vi "Arrange.vi"(6 "Variant in":variant, 7 "Shift Pressed?":bool, 8 "error in (no error)":errorcluster, 10 "QD Combo Box Ref":refnum<vi>, 11 "QD Launch VI Ref":refnum<vi>) -> (0 "error out":errorcluster, 4 "Variant out":variant)   [LabVIEW 2019]
doc: "Arranges the block diagram or front panel objects depending on the selection:\n\nFP + No Selection:\n Arranges all controls and indicators by relative position, snaps to grid and resets the panel origins.\n\nFP + Selection:\n Arranges the selected controls by the left edge and snaps to grid. \n Hold Shift to arrange the selected controls by the top edge.\n\nBD + No Selection:\n Arranges all terminals to the adjacent terminal and align controls/indicators left/right respectively.\n\nBD + Selection:\n Arranges the selected objects to adjacent terminal (left-to-right). \n Hold Shift to arrange the selection in reverse order (right-to-left).\n Note: Constants are arranged relative to the adjacent terminal position.\n\nCreated by: Ryan Pacini\n\nDefault Shortcut - [A]"
uses:
  _Script/support/_builtins_arrange.ctl
  _Script/support/Script.lvlib
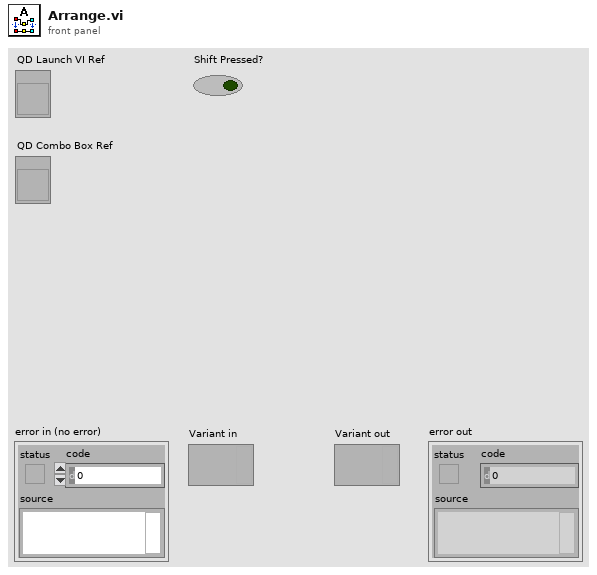
[diagram p1: front panel]
types:
  T1 = typedef "Script.lvlib/_builtins_arrange.ctl" = enum8{"left_to_right", "right_to_left"}
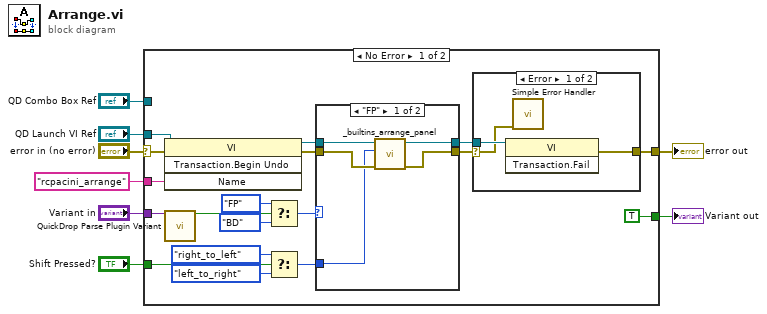
[diagram p0: block diagram]
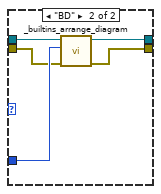
[diagram p2: hidden frame]
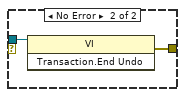
[diagram p3: hidden frame]
diagram:
  n1 = case shown="No Error" "error in (no error)" {
    selector: "error in (no error)" -> [w26 w42]
    tunnel: [w25 w42] -> w3
    tunnel: "QD Launch VI Ref" -> [w21 _]
    tunnel: "rcpacini_arrange" ("Undo Name") -> [w24 _]
    tunnel: "Variant in" -> [w22 _]
    tunnel: [TRUE _] -> w4
    tunnel: "QD Combo Box Ref" -> [_ _]
    tunnel: "Shift Pressed?" -> [w16 _]
    frame No Error {
      n2 = invoke class="VI" method="Transaction.Begin Undo"(reference=w21, error in=w26, "Name"=w24) -> (reference out=w20:refnum<vi>, error out=w19:errorcluster)  [unwired: 1 in, 2 out]
      n3 = call <vilib>:"QuickDrop Parse Plugin Variant.vi"("QDKS Variant in"=w22) -> ("QD Launch VI Panel?"=w12:bool)  [unwired: 12 in, 2 out]
      n4 = Select(t=enum8{"FP", "BD"}."FP" ("Panel"), s=w12, f=enum8{"FP", "BD"}."BD" ("Panel")) -> (s? t:f=w11:enum8{"FP", "BD"})
      n5 = Select(t=_builtins_arrange."right_to_left" ("Arrange"), s=w16, f=_builtins_arrange."left_to_right" ("Arrange")) -> (s? t:f=w15:T1)
      n6 = case shown="\"FP\"" w11 {
        tunnel: w20 -> [w28 w33]
        tunnel: w19 -> [w30 w32]
        tunnel: [w31 w36] -> w18
        tunnel: [w29 w35] -> w17
        tunnel: w15 -> [w27 w34]
        frame "FP" {
          n7 = call "_builtins_arrange_panel.vi"("error in (no error)"=w30, "Arrange"=w27, "VI Refnum in"=w28) -> ("error out"=w31:errorcluster, "VI Refnum out"=w29:refnum<vi>)  [unwired: 7 in]
        }
        frame "BD" {
          n8 = call "_builtins_arrange_diagram.vi"("error in (no error)"=w32, "Arrange"=w34, "VI Refnum in"=w33) -> ("error out"=w36:errorcluster, "VI Refnum out"=w35:refnum<vi>)  [unwired: 7 in]
        }
      }
      n9 = case shown="Error" w18 {
        selector: w18 -> [w37 _]
        tunnel: w17 -> [w38 w40]
        tunnel: [w39 w41] -> w25
        frame Error {
          n10 = invoke class="VI" method="Transaction.Fail"(reference=w38) -> (error out=w39:errorcluster)  [unwired: 2 in, 2 out]
          n11 = call <vilib>:"Simple Error Handler.vi"("error in (no error)"=w37) -> ()  [unwired: 4 in, 5 out]
        }
        frame No Error {
          n12 = invoke class="VI" method="Transaction.End Undo"(reference=w40) -> (error out=w41:errorcluster)  [unwired: 2 in, 2 out]
        }
      }
    }
    frame Error {
    }
  }
  "error out" <- w3
  "Variant out" <- w4
